vi "Get Alg.vi"(8 "error in (no error)":errorcluster, 11 "JWT in":refnum<class "JWT.lvclass">) -> (0 "error out":errorcluster, 2 "Signature Algorithm":T1, 3 "JWT out":refnum<class "JWT.lvclass">)   [LabVIEW 2017, in "JWT.lvlib" / "JWT.lvclass"]
uses:
  JWT.lvclass
  Signature Algorithms.ctl
  JWT.lvlib
  lv-json/JSON/JSON.lvlib
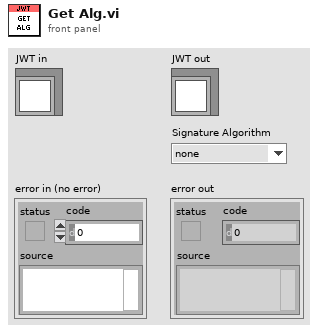
[diagram p1: front panel]
types:
  T1 = typedef "JWT.lvlib/Signature Algorithms.ctl" = enum16{"none", "HS256"}
  T2 = typedef "JSON.lvlib/JSON Item Type.ctl" = enum16{"unknown", "null", "Array", "Object", "String", "Number", "Boolean"}
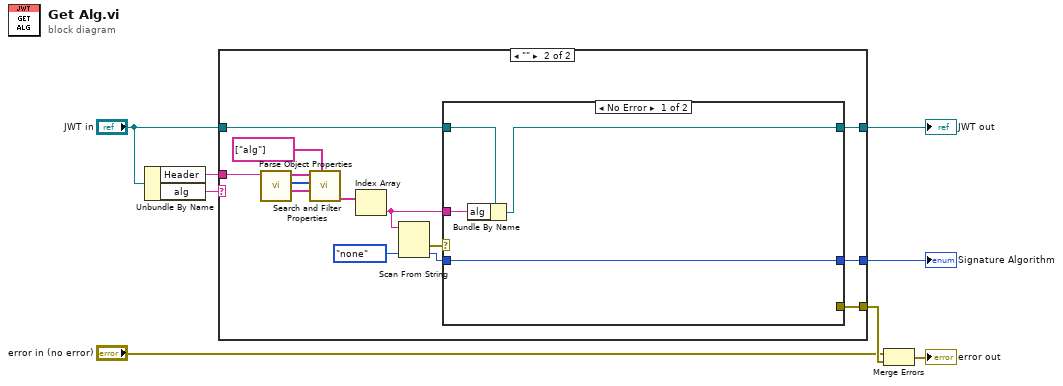
[diagram p0: block diagram]
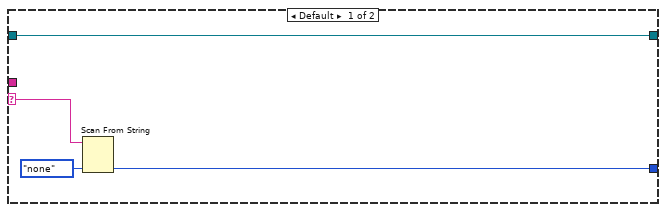
[diagram p2: hidden frame]
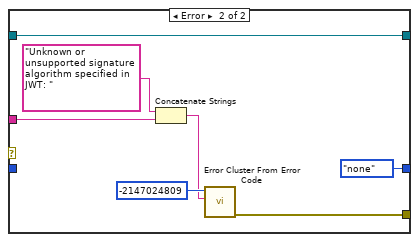
[diagram p3: hidden frame]
diagram:
  n1 = Unbundle By Name("JWT in") -> ("Header"=w8:string, "alg"=w1:string)
  n2 = case shown="\"\"" w1 {
    selector: w1 -> [w11 _]
    tunnel: w8 -> [_ w26]
    tunnel: [w10 w17] -> w7
    tunnel: [_ w16] -> w6
    tunnel: "JWT in" -> [w12 w15]
    tunnel: [w12 w14] -> w2
    frame Default {
      n3 = Scan From String(input string=w11, default 1=Signature_Algorithms."none" ("Signature Algorithms")) -> (output 1=w10:T1)  [unwired: 3 in, 3 out]
    }
    frame "" {
      n4 = call "Parse Object Properties.vi"("JSON String"=w26) -> ("Values"=w23:string[], "Item Types"=w24:T2[], "Keys"=w25:string[])  [unwired: 7 in, 1 out]
      n5 = call "Search and Filter Properties.vi"("Search Keys"=string[] ["alg"], "Values In"=w23, "Types In"=w24, "Keys In"=w25) -> ("Filtered Values"=w21:string[])  [unwired: 2 in, 5 out]
      n6 = Index Array(array=w21) -> (element=w13:string)  [unwired: 1 in]
      n7 = Scan From String(input string=w13, default 1=Signature_Algorithms."none" ("Signature Algorithms")) -> (error out=w19:errorcluster, output 1=w18:T1)  [unwired: 3 in, 2 out]
      n8 = case shown="No Error" w19 {
        tunnel: w13 -> [w27 w34]
        tunnel: w18 -> [w28 _]
        tunnel: [w28 Signature_Algorithms."none" ("Signature Algorithms")] -> w17
        tunnel: [_ w33] -> w16
        tunnel: w15 -> [w30 w31]
        tunnel: [w29 w31] -> w14
        frame No Error {
          n9 = Bundle By Name(cluster=w30, "alg"=w27) -> (w29:refnum<class "JWT.lvclass">)
        }
        frame Error {
          n10 = Concatenate Strings("Unknown or unsupported signature algorithm specified in JWT: ", w34) -> (w32:string)
          n11 = call <vilib>:"Error Cluster From Error Code.vi"("error message (\"\")"=w32, "error code (0)"=-2147024809) -> ("error out"=w33:errorcluster)  [unwired: 7 in]
        }
      }
    }
  }
  "JWT out" <- w2
  "Signature Algorithm" <- w7
  n12 = Merge Errors("error in (no error)", w6) -> (→"error out":errorcluster)
